vi "openDB.vi"(0 "Open Button":bool) -> (1 "standard output":string, 2 "error out":errorcluster)   [LabVIEW 2015]
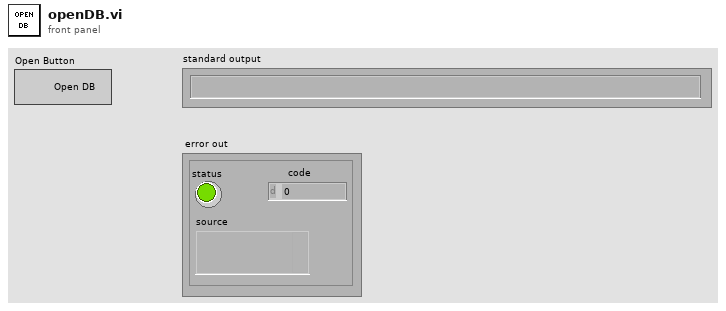
[diagram p1: front panel]
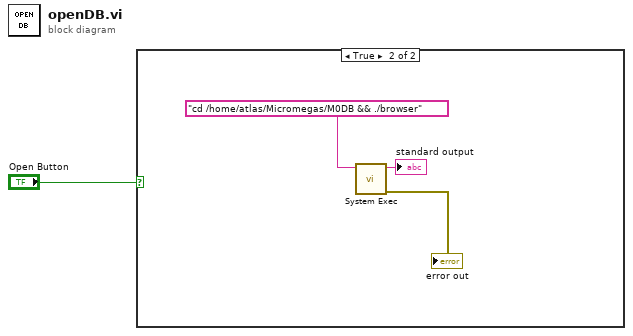
[diagram p0: block diagram]
diagram:
  n1 = case shown="True" "Open Button" {
    frame False {
    }
    frame True {
      n2 = call <vilib>:"System Exec.vi"("command line"="cd /home/atlas/Micromegas/M0DB && ./browser") -> ("error out"=→"error out":errorcluster, "standard output"=→"standard output":string)  [unwired: 7 in, 2 out]
    }
  }
